vi "GetOverlay.vi"(8 "error in":errorcluster, 11 "NISE_CEF_serializable node in":refnum<class "NISE_CEF_serializable node.lvclass">) -> (0 "error out":errorcluster, 2 "overlay":string, 3 "NISE_CEF_serializable node out":refnum<class "NISE_CEF_serializable node.lvclass">)   [LabVIEW 2013, in "NISE_CEF_serializable node.lvclass"]
uses:
  NISE_CEF_serializable node.lvclass
  serializable configuration/NISE_CEF_serializable configuration.lvclass
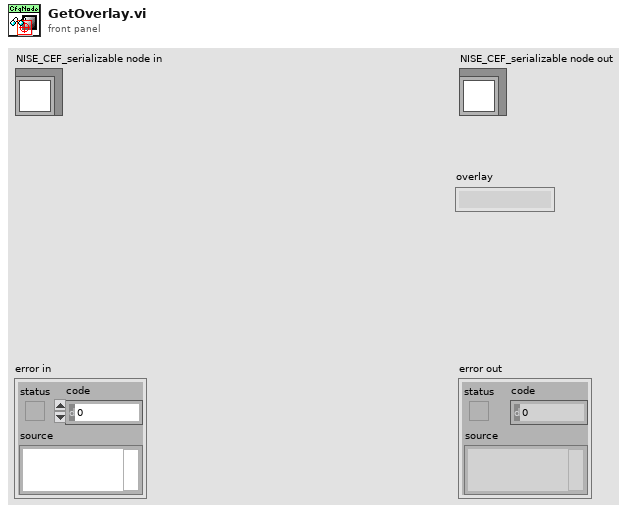
[diagram p1: front panel]
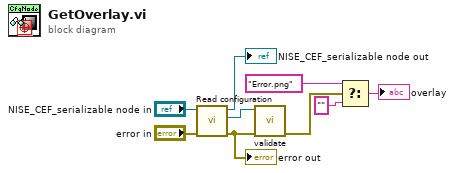
[diagram p0: block diagram]
diagram:
  n1 = call-dynamic "Read configuration.vi"("error in"="error in", "NISE_CEF_serializable node in"="NISE_CEF_serializable node in") -> ("error out"=w4:errorcluster, "configuration"=w5:refnum<class "NISE_CEF_serializable configuration.lvclass">, "NISE_CEF_serializable node out"=→"NISE_CEF_serializable node out":refnum<class "NISE_CEF_serializable node.lvclass">)  [unwired: 7 in]
  "error out" <- w4
  n2 = call-dynamic "validate.vi"("error in"=w4, "configuration in"=w5) -> ("error out"=w3:errorcluster)  [unwired: 8 in, 1 out]
  n3 = Select(t="Error.png", s=w3, f="") -> (s? t:f=→"overlay":string)
